vi "Sinus While Loop.vi"() -> ()   [LabVIEW 2014]
uses:
  Documents/LabVIEW Data/Unbenanntes Projekt 8/support/Message Queue/Message Cluster.ctl
  All Message Queues.ctl
  state machine enum.ctl
  Documents/LabVIEW Data/Unbenanntes Projekt 8/support/Message Queue/Enqueue Message (Single).vi
  Documents/LabVIEW Data/Unbenanntes Projekt 8/support/Message Queue/Message Queue.lvlib
panel:
  out "Aktuelle Position":string
  out "Status":string
  in  "Nachrichten-Queues (Ausgang)":T1
  out "Numerisch":i32
  out "Elemente":T2[](array[typedef])
  in  "StartErf":bool
  in  "StoppErf":bool
  in  "StoppM":bool
  in  "StartM":bool
  out "Signalverlaufsdiagramm":dbl(graph)
  out "i 3":i32
  out "Motor verfährt":bool
  out "Fehler (Ausgang)":errorcluster
  in  "Exit":bool
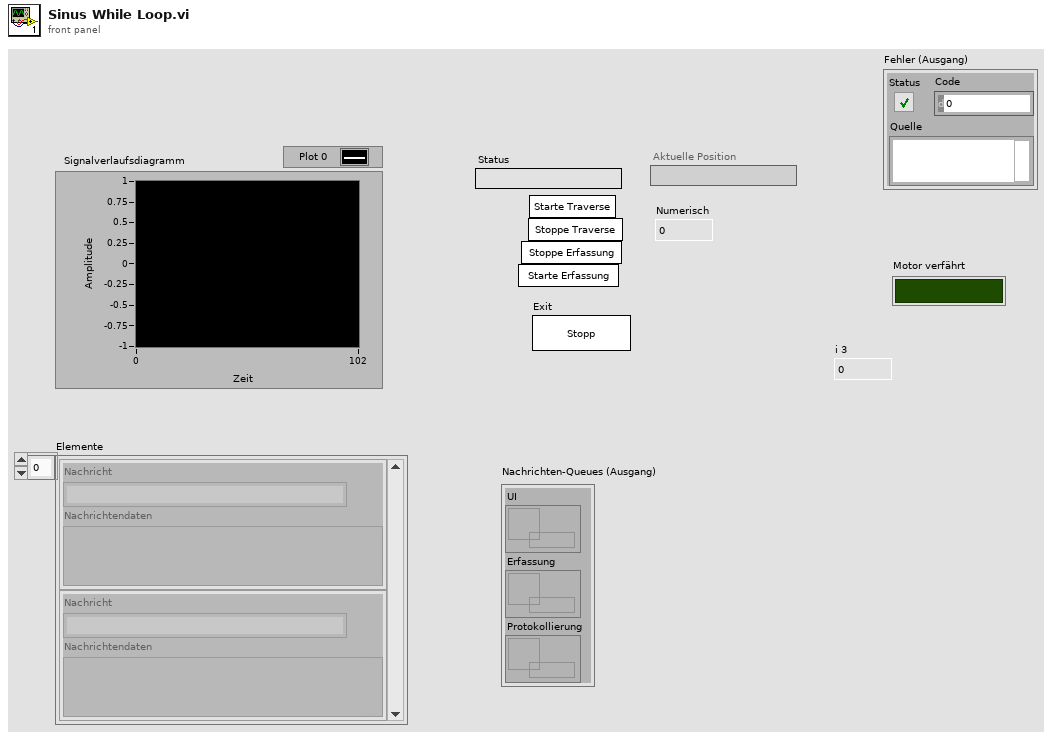
[diagram p1: front panel]
types:
  T1 = typedef "Message Queue.lvlib/All Message Queues.ctl" = cluster{"UI":refnum<queue>, "Erfassung":refnum<queue>, "Traverse":refnum<queue>}
  T2 = typedef "Message Queue.lvlib/Message Cluster.ctl" = cluster{"Nachricht":string, "Nachrichtendaten":variant}
  T3 = typedef "state machine enum.ctl" = enum16{"Stopp", "Wartet auf Eingaben", "Exit", "Start", "Traverse x Messwerte"}
  T4 = cluster{"Status":bool, "Code":i32, "Quelle":string}
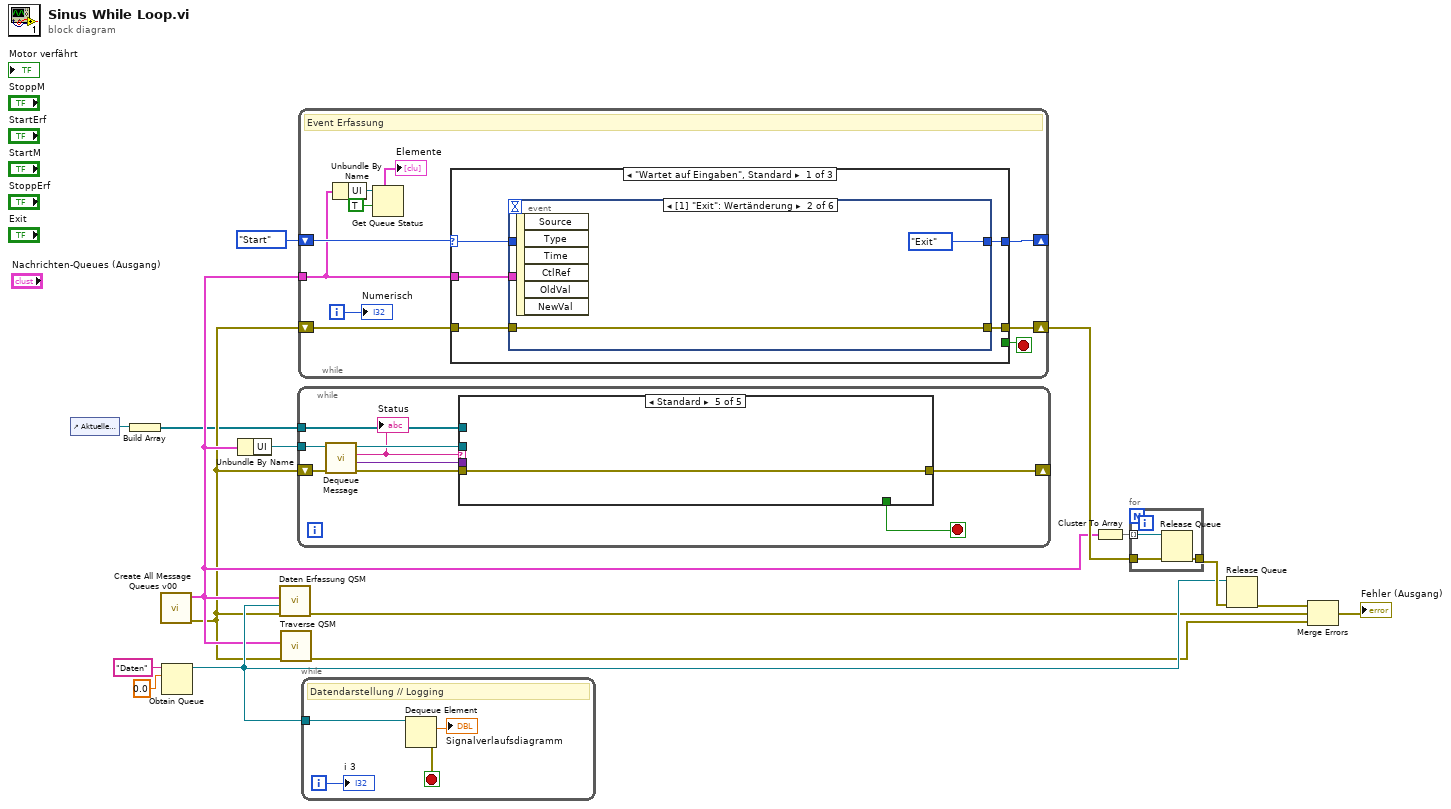
[diagram p0: block diagram]
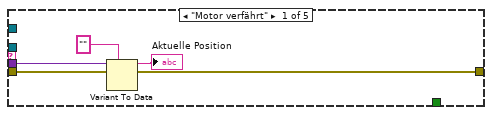
[diagram p2: hidden frame]
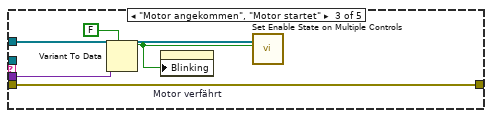
[diagram p4: hidden frame]
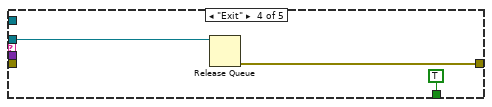
[diagram p5: hidden frame]
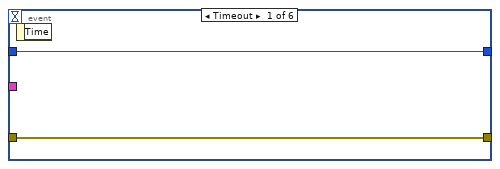
[diagram p6: hidden frame]
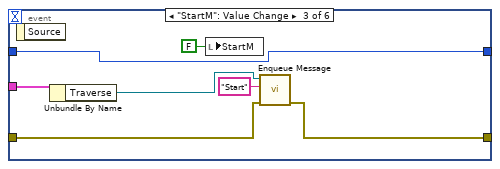
[diagram p7: hidden frame]
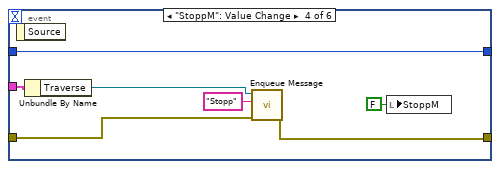
[diagram p8: hidden frame]
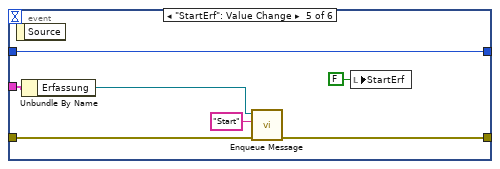
[diagram p9: hidden frame]
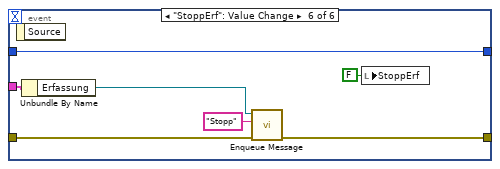
[diagram p10: hidden frame]
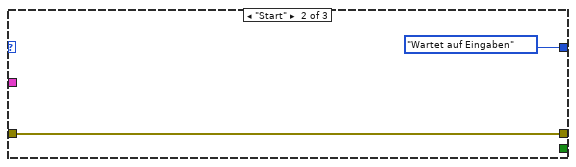
[diagram p11: hidden frame]
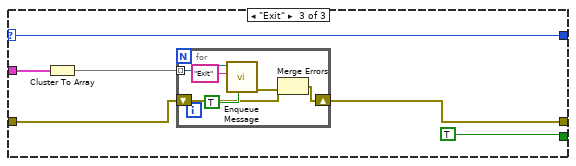
[diagram p12: hidden frame]
diagram:
  n1 = control-ref of="Aktuelle Position"() -> (w2:refnum<vi>)
  n2 = Build Array(w2) -> (w1:refnum<vi>[])
  n3 = call "Create All Message Queues v00.vi"() -> ("error out"=w3:T4, "Nachrichten-Queues (Ausgang)"=w5:T1)  [unwired: 10 in]
  n4 = Obtain Queue(name (unnamed)="Daten" ("Name (unbenannt)"), element data type=0.0) -> (queue out=w8:refnum<queue>)  [unwired: 3 in, 2 out]
  n5 = Unbundle By Name(w5) -> ("UI"=w4:refnum<queue>)
  n6 = call "Daten Erfassung QSM.vi"("error in"=w3, "Daten-Queue (Eingang)"=w8, "Nachrichten-Queues (Eingang)"=w5) -> ("error out"=w7:errorcluster)  [unwired: 8 in]
  n7 = call "Traverse QSM.vi"("error in"=w3, "Nachrichten-Queues (Eingang)"=w5) -> ("error out"=w6:errorcluster)  [unwired: 9 in]
  n8 = while {
    tunnel: w4 -> [w25]
    shift-right: [w20] -> _
    shift-left: w3 -> [w21]
    tunnel: w1 -> [w18]
    stop <- w17 stop-if-true
    n9 = call "Dequeue Message.vi"("error in (no error)"=w21, "Nachrichten-Queue"=w25) -> ("error out"=w22:T4, "Nachrichtendaten"=w23:variant, "Nachricht"=w19:string, "Nachrichten-Queue (Kopie)"=w24:refnum<queue>)  [unwired: 6 in]
    "Status" <- w19
    n10 = case shown="Standard" w19 {
      tunnel: w24 -> [_ _ _ w38 _]
      tunnel: w23 -> [w28 _ w34 _ _]
      tunnel: w22 -> [w29 w30 w35 _ w39]
      tunnel: [w29 w30 w35 w37 w39] -> w20
      tunnel: w18 -> [_ _ w32 _ _]
      tunnel: [_ _ _ TRUE _] -> w17
      frame "Motor verfährt" {
        n11 = Variant To Data(type="", Variant=w28) -> (data=→"Aktuelle Position":string)  [unwired: 1 in, 1 out]
      }
      frame "Initialize" {
      }
      frame "Motor angekommen", "Motor startet" {
        n12 = Variant To Data(type=FALSE ("Blinkend"), Variant=w34) -> (data=w31:bool)  [unwired: 1 in, 1 out]
        n13 = property on="Motor verfährt" class="Bool. (strikt)"("Blinking"=w31) -> ()  [unwired: 2 in, 2 out]
        n14 = call "Set Enable State on Multiple Controls.vi"("Aktivieren?"=w31, "Elemente"=w32) -> ()  [unwired: 10 in]
      }
      frame "Exit" {
        n15 = Release Queue(queue=w38) -> (error out=w37:errorcluster)  [unwired: 2 in, 2 out]
      }
      frame Default {
      }
    }
  }
  n16 = while {
    shift-right: [w48] -> _
    shift-left: state_machine_enum."Start" -> [w49]
    tunnel: w5 -> [w42]
    shift-right: [w47] -> w12
    shift-left: w3 -> [w46]
    i -> [w41]
    stop <- w45 stop-if-true
    # "Event Erfassung"
    n17 = Unbundle By Name(w42) -> ("UI"=w43:refnum<queue>)
    n18 = Get Queue Status(queue=w43, return elements? (F)=TRUE ("Elemente ausgeben? (F)")) -> (elements=→"Elemente":T2[])  [unwired: 1 in, 7 out]
    n19 = case shown="\"Wartet auf Eingaben\", Standard" w49 {
      selector: w49 -> [w51 _ w92]
      tunnel: [w54 state_machine_enum."Wartet auf Eingaben" w92] -> w48
      tunnel: w42 -> [w53 _ w90]
      tunnel: [w52 w87 w94] -> w47
      tunnel: w46 -> [w50 w87 w93]
      tunnel: [_ _ TRUE] -> w45
      frame "Wartet auf Eingaben", Default {
        n20 = event shown="[1] \"Exit\": Wertänderung" {
          selector: _ -> [_ _ _ _ _ _]
          dyn-events: _ -> [_ _ _ _ _ _]
          timeout: _ -> [_ _ _ _ _ _]
          tunnel: [w56 state_machine_enum."Exit" w59 w68 w75 w82] -> w54
          tunnel: w53 -> [_ _ w64 w71 w78 w85]
          tunnel: [w55 w57 w62 w69 w76 w83] -> w52
          tunnel: w51 -> [w56 _ w59 w68 w75 w82]
          tunnel: w50 -> [w55 w57 w61 w67 w74 w81]
          event Timeout {
            n21 = event-data() -> ()  [unwired: 1 in, 1 out]
          }
          event "Exit": Value Change {
            n22 = event-data() -> ()  [unwired: 1 in, 6 out]
          }
          event "StartM": Value Change {
            n23 = event-data() -> ()  [unwired: 1 in, 1 out]
            n24 = Unbundle By Name(w64) -> ("Traverse"=w63:refnum<queue>)
            n25 = local write "StartM"(FALSE ("StartM")) -> ()
            n26 = call-poly "Enqueue Message.vi"("error in (no error)"=w61, "Nachricht"="Start", "Nachrichten-Queue"=w63) -> ("error out"=w62:T4)  [unwired: 7 in, 1 out]
          }
          event "StoppM": Value Change {
            n27 = event-data() -> ()  [unwired: 1 in, 1 out]
            n28 = Unbundle By Name(w71) -> ("Traverse"=w70:refnum<queue>)
            n29 = call-poly "Enqueue Message.vi"("error in (no error)"=w67, "Nachricht"="Stopp", "Nachrichten-Queue"=w70) -> ("error out"=w69:T4)  [unwired: 7 in, 1 out]
            n30 = local write "StoppM"(FALSE ("StartM")) -> ()
          }
          event "StartErf": Value Change {
            n31 = event-data() -> ()  [unwired: 1 in, 1 out]
            n32 = Unbundle By Name(w78) -> ("Erfassung"=w77:refnum<queue>)
            n33 = call-poly "Enqueue Message.vi"("error in (no error)"=w74, "Nachricht"="Start", "Nachrichten-Queue"=w77) -> ("error out"=w76:T4)  [unwired: 7 in, 1 out]
            n34 = local write "StartErf"(FALSE ("StartM")) -> ()
          }
          event "StoppErf": Value Change {
            n35 = event-data() -> ()  [unwired: 1 in, 1 out]
            n36 = Unbundle By Name(w85) -> ("Erfassung"=w84:refnum<queue>)
            n37 = call-poly "Enqueue Message.vi"("error in (no error)"=w81, "Nachricht"="Stopp", "Nachrichten-Queue"=w84) -> ("error out"=w83:T4)  [unwired: 7 in, 1 out]
            n38 = local write "StoppErf"(FALSE ("StartM")) -> ()
          }
        }
      }
      frame "Start" {
      }
      frame "Exit" {
        n39 = Cluster To Array(cluster=w90) -> (array=w89:refnum<queue>[])
        n40 = for {
          tunnel: w89 -> [w99] mode=indexing
          shift-right: [w96] -> w94
          shift-left: w93 -> [w95]
          n41 = call-poly "Enqueue Message.vi"("Nachricht mit Priorität? (F)"=TRUE, "Nachricht"="Exit", "Nachrichten-Queue"=w99) -> ("error out"=w97:T4)  [unwired: 7 in, 1 out]
          n42 = Merge Errors(w95, w97) -> (w96:errorcluster)
        }
      }
    }
    "Numerisch" <- w41
  }
  n43 = while {
    tunnel: w8 -> [w103]
    i -> [w104]
    stop <- w101 stop-if-true
    # "Datendarstellung // Logging"
    n44 = Dequeue Element(queue=w103) -> (element=→"Signalverlaufsdiagramm":dbl, error out=w101:errorcluster)  [unwired: 2 in, 2 out]
    "i 3" <- w104
  }
  n45 = Cluster To Array(cluster=w5) -> (array=w13:refnum<queue>[])
  n46 = for {
    tunnel: w13 -> [w107] mode=indexing
    tunnel: [w106] -> w11
    tunnel: w12 -> [w105]
    n47 = Release Queue(queue=w107, error in (no error)=w105) -> (error out=w106:errorcluster)  [unwired: 1 in, 2 out]
  }
  n48 = Release Queue(queue=w8, error in (no error)=w11) -> (error out=w10:errorcluster)  [unwired: 1 in, 2 out]
  n49 = Merge Errors(w10, w7, w6) -> (→"Fehler (Ausgang)":errorcluster)
